vi "Actor Teardown Core.vi"(7 "Actor":refnum<class "Actor.lvclass">, 10 "Error":errorcluster, 11 "Msging Self Actor State in":refnum<class "Msging Self Actor State.lvclass">) -> (0 "error out":errorcluster, 2 "Teardown?":bool)   [LabVIEW 2021, in "jettl.lvlib" / "Msging Self Actor State.lvclass"]
uses:
  Msging Self Actor State.lvclass
  Actor/Actor.lvclass
  Msgs/Actor Destroy/Actor Destroy Msg Strategy/Actor Destroy Msg Strategy.lvclass
  C:/git/jettl/src/LVCAM/LVCAM/Msg Strategy/Msg Strategy.lvclass
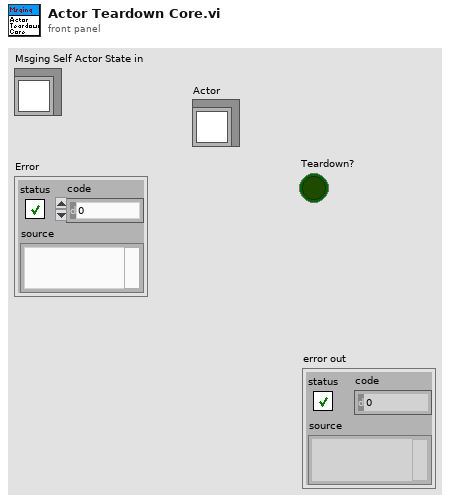
[diagram p1: front panel]
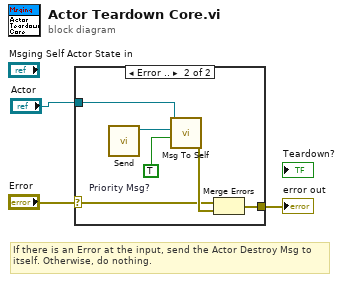
[diagram p0: block diagram]
diagram:
  # "If there is an Error at the input, send the Actor Destroy Msg to itself. Otherwise, do nothing."
  n1 = case shown="Error .." "Error" {
    selector: "Error" -> [_ w4]
    tunnel: [_ w9] -> w2
    tunnel: "Actor" -> [_ w8]
    frame No Error {
    }
    frame Error {
      w6 = TRUE  # Priority Msg?
      n2 = call "Send.vi"() -> ("Actor Destroy Msg Strategy out"=w7:refnum<class "Actor Destroy Msg Strategy.lvclass">)  [unwired: 11 in]
      n3 = call-dynamic "Msg To Self.vi"("Priority Msg?"=w6, "Msg"=w7, "Actor in"=w8) -> ("error out"=w5:errorcluster)  [unwired: 8 in]
      n4 = Merge Errors(w4, w5) -> (w9:errorcluster)
    }
  }
  "error out" <- w2
